vi "Write Series.vi"(8 "error in (no error)":errorcluster, 10 "Series":T1(ring), 11 "Astromech droid in":refnum<class "Astromech droid.lvclass">) -> (0 "error out":errorcluster, 3 "Astromech droid out":refnum<class "Astromech droid.lvclass">)   [LabVIEW 2021, in "Astromech droid.lvclass"]
uses:
  Astromech droid.lvclass
  Astromech droid.lvclass/Astromech droid.ctl
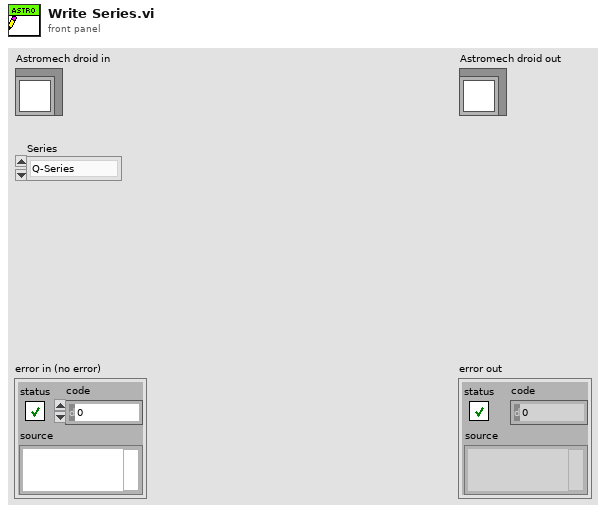
[diagram p1: front panel]
types:
  T1 = enum16{"Q-Series", "BB-Series", "C-Series", "R-Series"}
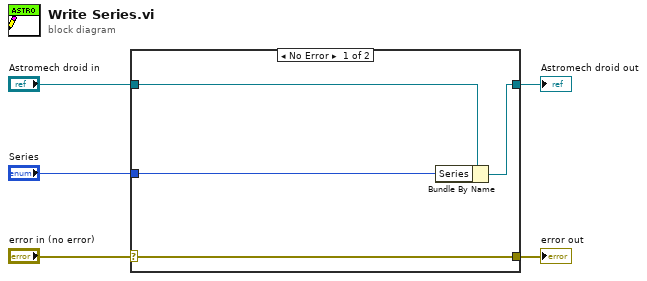
[diagram p0: block diagram]
diagram:
  n1 = case shown="No Error" "error in (no error)" {
    selector: "error in (no error)" -> [w9 w10]
    tunnel: [w9 w10] -> w4
    tunnel: [w7 w11] -> w2
    tunnel: "Astromech droid in" -> [w8 w11]
    tunnel: "Series" -> [w6 _]
    frame No Error {
      n2 = Bundle By Name(cluster=w8, "Series"=w6) -> (w7:refnum<class "Astromech droid.lvclass">)
    }
    frame Error {
    }
  }
  "error out" <- w4
  "Astromech droid out" <- w2
